vi "Slack-Get Bot Channel.vi"(0 "config in":T1, 11 "error in (no error)":errorcluster) -> (4 "config out":T1, 15 "error out":errorcluster)   [LabVIEW 2015]
uses:
  Typedefs/Slack-Configuration.ctl
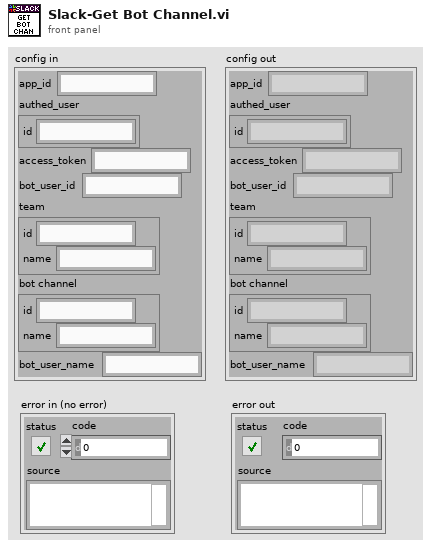
[diagram p1: front panel]
types:
  T1 = typedef "Slack-Configuration.ctl" = cluster{"app_id":string, "authed_user":cluster{"id":string}, "access_token":string, "bot_user_id":string, "team":cluster{"id":string, "name":string}, "bot channel":cluster{"id":string, "name":string}, "bot_user_name":string}
  T2 = cluster{"channels":cluster{"id":string, "name":string, "is_channel":bool}[]}
  T3 = typedef "Slack-User.ctl" = cluster{"id":string, "name":string}
  T4 = cluster{"id":string, "name":string, "is_channel":bool}[]
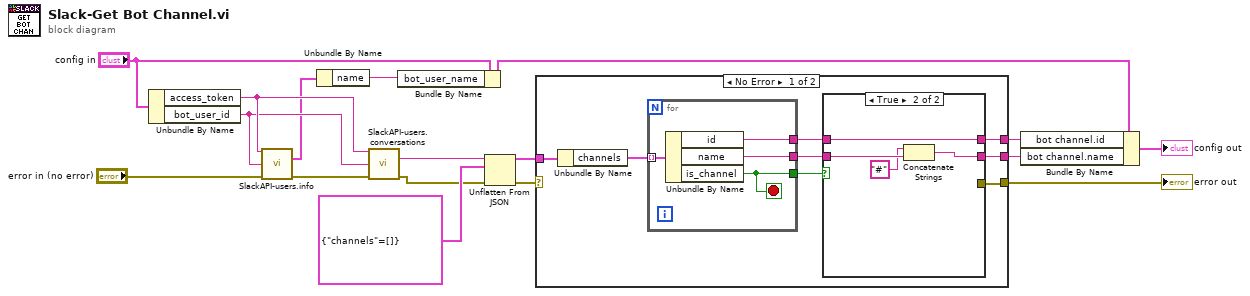
[diagram p0: block diagram]
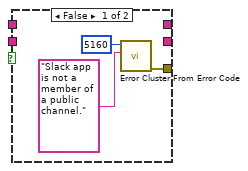
[diagram p2: hidden frame]
diagram:
  n1 = Unbundle By Name("config in") -> ("access_token"=w5:string, "bot_user_id"=w4:string)
  n2 = call "SlackAPI-users.info.vi"("token"=w5, "user"=w4, "error in (no error)"="error in (no error)") -> ("user"=w2:T3, "error out"=w6:errorcluster)  [unwired: 10 in, 1 out]
  n3 = Unbundle By Name(w2) -> ("name"=w1:string)
  n4 = call "SlackAPI-users.conversations.vi"("token"=w5, "user"=w4, "error in (no error)"=w6) -> ("body"=w16:string, "error out"=w15:errorcluster)  [unwired: 10 in, 1 out]
  n5 = Bundle By Name(cluster="config in", "bot_user_name"=w1) -> (w3:T1)
  n6 = Unflatten From JSON(JSON string=w16, type and defaults=T2 {"channels"=[]} ("Cluster"), error in (no error)=w15) -> (value=w14:T2, error out=w13:errorcluster)  [unwired: 4 in]
  n7 = case shown="No Error" w13 {
    selector: w13 -> [_ w37]
    tunnel: w14 -> [w25 _]
    tunnel: [w20 w37] -> w12
    tunnel: [w19 _] -> w9
    tunnel: [w18 _] -> w8
    frame No Error {
      n8 = Unbundle By Name(w25) -> ("channels"=w24:T4)
      n9 = for {
        tunnel: w24 -> [w36] mode=indexing
        tunnel: [w35] -> w22
        tunnel: [w34] -> w21
        tunnel: [w33] -> w23
        stop <- w33 stop-if-true
        n10 = Unbundle By Name(w36) -> ("id"=w35:string, "name"=w34:string, "is_channel"=w33:bool)
      }
      n11 = case shown="True" w23 {
        tunnel: w22 -> [_ w32]
        tunnel: w21 -> [_ w31]
        tunnel: [w28 _] -> w20
        tunnel: [_ w32] -> w19
        tunnel: [_ w30] -> w18
        frame False {
          n12 = call <vilib>:"Error Cluster From Error Code.vi"("error message (\"\")"="Slack app is not a member of a public channel.", "error code (0)"=5160) -> ("error out"=w28:errorcluster)  [unwired: 7 in]
        }
        frame True {
          n13 = Concatenate Strings("#", w31) -> (w30:string)
        }
      }
    }
    frame Error {
    }
  }
  "error out" <- w12
  n14 = Bundle By Name(cluster=w3, "bot channel.id"=w9, "bot channel.name"=w8) -> (→"config out":T1)
